vi "manage loss communication.vi"(8 "error in (no error)":errorcluster, 11 "Channel in":refnum<class "Channel.lvclass">) -> (0 "error out":errorcluster, 3 "Channel out":refnum<class "Channel.lvclass">)   [LabVIEW 2018, in "Channel.lvclass"]
uses:
  Channel.lvclass
  Channel.lvclass/Channel.ctl
  Header content/Header content.lvclass/Header content.ctl
  Server/Server.lvclass
  Log File/CCS_Log File.lvclass
  Header content/Header content.lvclass
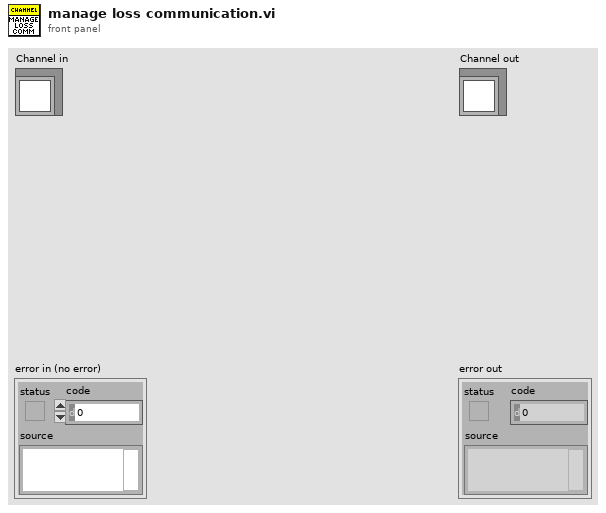
[diagram p1: front panel]
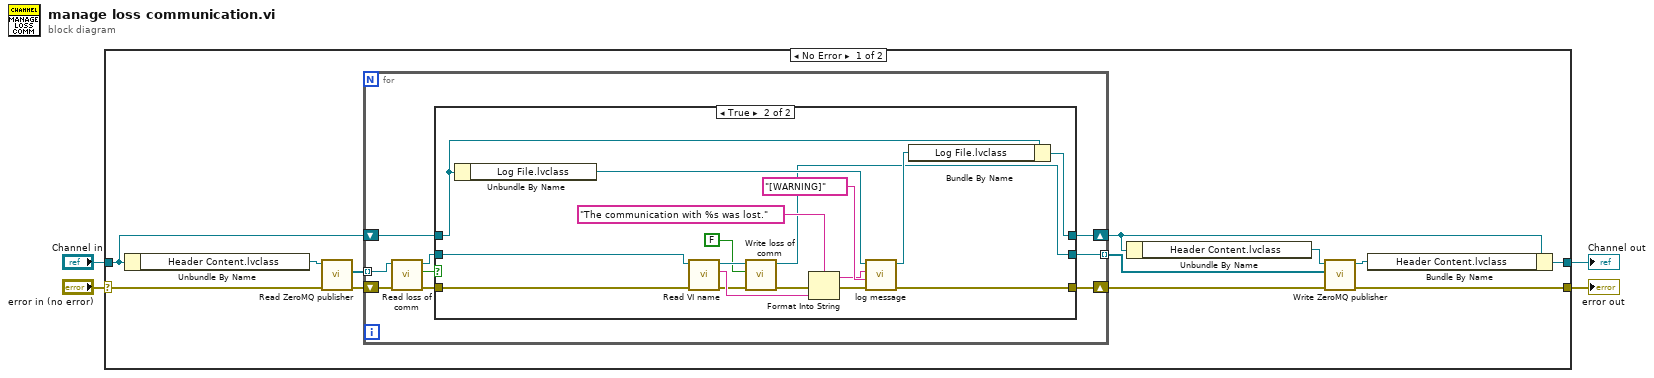
[diagram p0: block diagram]
diagram:
  n1 = case shown="No Error" "error in (no error)" {
    selector: "error in (no error)" -> [w12 w47]
    tunnel: [w6 w47] -> w3
    tunnel: [w5 w46] -> w1
    tunnel: "Channel in" -> [w13 w46]
    frame No Error {
      n2 = Unbundle By Name(w13) -> ("Header Content.lvclass"=w16:refnum<class "Header content.lvclass">)
      n3 = call "Read ZeroMQ publisher.vi"("error in (no error)"=w12, "Header content in"=w16) -> ("error out"=w14:errorcluster, "ZeroMQ publisher"=w15:refnum<class "Server.lvclass">[])  [unwired: 7 in, 1 out]
      n4 = for {
        shift-right: [w24] -> w8
        shift-left: w13 -> [w25]
        shift-right: [w23] -> w11
        shift-left: w14 -> [w20]
        tunnel: w15 -> [w21] mode=indexing
        tunnel: [w17] -> w10 mode=indexing
        n5 = call-dynamic "Read loss of comm.vi"("error in (no error)"=w20, "Server in"=w21) -> ("error out"=w19:errorcluster, "loss of comm"=w18:bool, "Server out"=w22:refnum<class "Server.lvclass">)  [unwired: 7 in]
        n6 = case shown="True" w18 {
          tunnel: w25 -> [w28 w45]
          tunnel: [w28 w44] -> w24
          tunnel: [w27 w43] -> w23
          tunnel: w22 -> [w26 w39]
          tunnel: w19 -> [w27 w38]
          tunnel: [w26 w29] -> w17
          frame False {
          }
          frame True {
            n7 = Unbundle By Name(w45) -> ("Log File.lvclass"=w42:refnum<class "CCS_Log File.lvclass">)
            n8 = call-dynamic "Read VI name.vi"("error in (no error)"=w38, "Server in"=w39) -> ("error out"=w33:errorcluster, "VI name"=w35:string, "Server out"=w31:refnum<class "Server.lvclass">)  [unwired: 7 in]
            n9 = call-dynamic "Write loss of comm.vi"("error in (no error)"=w33, "loss of comm"=FALSE, "Server in"=w31) -> ("error out"=w32:errorcluster, "Server out"=w29:refnum<class "Server.lvclass">)  [unwired: 7 in]
            n10 = Format Into String(format string="The communication with %s was lost.", error in=w32, w35) -> (resulting string=w37:string, error out=w36:errorcluster)  [unwired: 1 in]
            n11 = call-dynamic "log message.vi"("error in (no error)"=w36, "message type"="[WARNING]", "Message to log"=w37, "Log File in"=w42) -> ("error out"=w43:errorcluster, "Log File out"=w41:refnum<class "CCS_Log File.lvclass">)  [unwired: 6 in]
            n12 = Bundle By Name(cluster=w45, "Log File.lvclass"=w41) -> (w44:refnum<class "Channel.lvclass">)
          }
        }
      }
      n13 = Unbundle By Name(w8) -> ("Header Content.lvclass"=w9:refnum<class "Header content.lvclass">)
      n14 = call-dynamic "Write ZeroMQ publisher.vi"("error in (no error)"=w11, "ZeroMQ publisher"=w10, "Header content in"=w9) -> ("error out"=w6:errorcluster, "Header content out"=w7:refnum<class "Header content.lvclass">)  [unwired: 7 in]
      n15 = Bundle By Name(cluster=w8, "Header Content.lvclass"=w7) -> (w5:refnum<class "Channel.lvclass">)
    }
    frame Error {
    }
  }
  "error out" <- w3
  "Channel out" <- w1
